vi "bytes at port reading count (subVI).vi"(0 "VISA Refnum in":refnum<visa-resource-name>, 1 "error in (no error)":errorcluster) -> (2 "VISA resource name out":refnum<visa-resource-name>, 3 "bytes read":u32, 4 "error out":errorcluster)   [LabVIEW 2016]
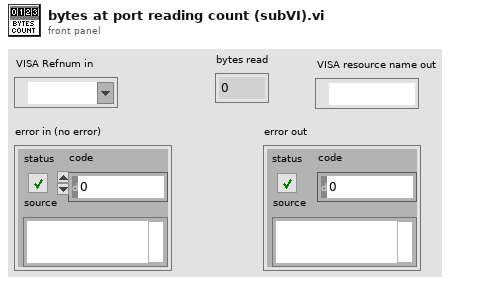
[diagram p1: front panel]
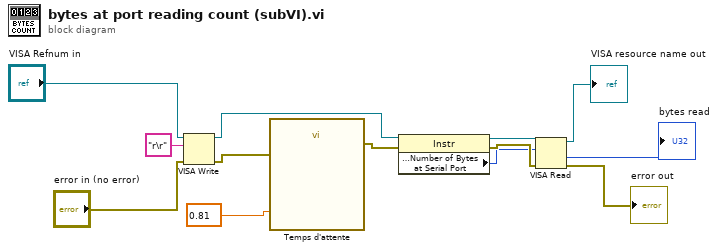
[diagram p0: block diagram]
diagram:
  n1 = VISA Write(VISA resource name="VISA Refnum in", write buffer="r\r" ("buffer d'écriture"), error in (no error)="error in (no error)") -> (VISA resource name out=w6:refnum<visa-resource-name>, error out=w7:errorcluster)  [unwired: 1 out]
  n2 = call "Temps d'attente"("error in (no error)"=w7, "Delay Time (s)"=0.81) -> ("error out"=w8:errorcluster)  [unwired: 9 in]
  n3 = property class="Instr"(reference=w6, error in=w8) -> (reference out=w9:refnum<visa-resource-name>, error out=w11:errorcluster, "Serial Settings:Number of Bytes at Serial Port"=w10:u32)
  n4 = VISA Read(VISA resource name=w9, byte count=w10, error in (no error)=w11) -> (VISA resource name out=→"VISA resource name out":refnum<visa-resource-name>, return count=→"bytes read":u32, error out=→"error out":errorcluster)  [unwired: 1 out]
